vi "Find_GT_File_Path.vi"(8 "error in":errorcluster, 10 "GT Mask Folder Path":path=path "D:/DNN/MVTec/pill/ground_truth", 11 "Image File Path":path=path "D:/DNN/MVTec/pill/ground_truth") -> (0 "error out":errorcluster, 1 "Found?":bool, 2 "GT File Path":path, 3 "Image File Path out":path=path "D:/DNN/MVTec/pill/ground_truth")   [LabVIEW 2024]
panel:
  out "Progress":i32
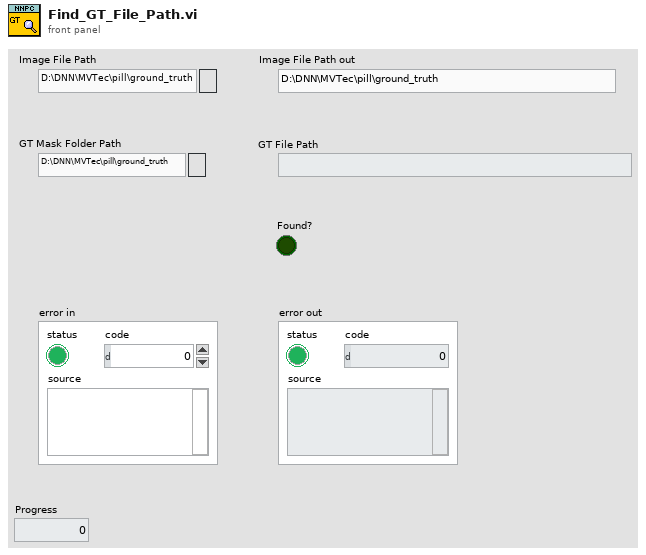
[diagram p1: front panel]
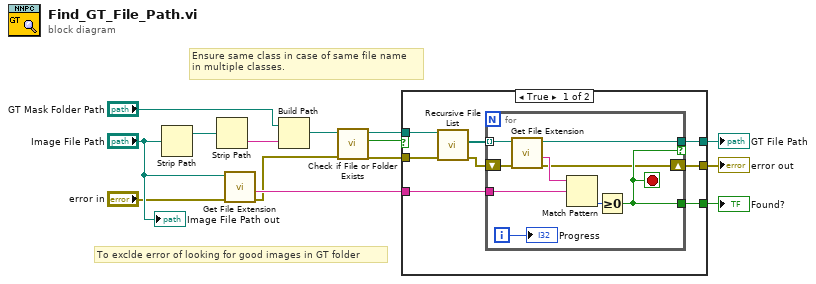
[diagram p0: block diagram]
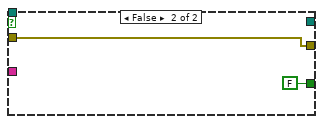
[diagram p2: hidden frame]
diagram:
  # "To exclde error of looking for good images in GT folder"
  # "Ensure same class in case of same file name\nin multiple classes."
  n1 = Strip Path(path="Image File Path") -> (stripped path=w14:path)  [unwired: 1 out]
  n2 = Strip Path(path=w14) -> (name=w13:string)  [unwired: 1 out]
  n3 = call <vilib>:"Get File Extension.vi"("error in (no error)"="error in", "file"="Image File Path") -> ("error out"=w6:errorcluster, "filename without extension"=w11:string)  [unwired: 5 in, 3 out]
  n4 = Build Path(base path="GT Mask Folder Path", name or relative path=w13) -> (appended path=w5:path)
  n5 = call <vilib>:"Check if File or Folder Exists.vi"("error in (no error)"=w6, "path"=w5) -> ("error out"=w3:errorcluster, "file or folder exists?"=w2:bool, "dup path"=w4:path)  [unwired: 7 in]
  n6 = case shown="True" w2 {
    tunnel: w11 -> [w22 _]
    tunnel: [w21 _] -> w10
    tunnel: [w20 FALSE] -> w9
    tunnel: [w17 w33] -> w8
    tunnel: w4 -> [w16 _]
    tunnel: w3 -> [w15 w33]
    frame True {
      n7 = call <vilib>:"Recursive File List.vi"("error in (no error)"=w15, "Folder Path"=w16) -> ("error out"=w18:errorcluster, "All Files in Dir"=w19:path[])  [unwired: 5 in, 3 out]
      n8 = for {
        tunnel: w19 -> [w28] mode=indexing
        tunnel: w22 -> [w31]
        tunnel: [w27] -> w21 if=w26
        tunnel: [w26] -> w20
        shift-right: [w24] -> w17
        shift-left: w18 -> [w25]
        i -> [w23]
        stop <- w26 stop-if-true
        n9 = call <vilib>:"Get File Extension.vi"("error in (no error)"=w25, "file"=w28) -> ("error out"=w24:errorcluster, "filename without extension"=w29:string, "dup file"=w27:path)  [unwired: 5 in, 2 out]
        n10 = Match Pattern(string=w29, regular expression=w31) -> (offset past match=w30:i32)  [unwired: 1 in, 3 out]
        n11 = Greater Or Equal To 0?(x=w30) -> (x >= 0?=w26:bool)
        "Progress" <- w23
      }
    }
    frame False {
    }
  }
  "GT File Path" <- w10
  "Found?" <- w9
  "error out" <- w8
  "Image File Path out" <- "Image File Path"
